vi "AUTON_Index.vi"(0 "Auton Array":dbl[][](array[numeric]), 5 "MeasuredHeading":dbl, 7 "LeftEncoder":dbl, 9 "RightEncoder":dbl, 11 "Harvester DIO":bool) -> (4 "Left Drive":dbl, 6 "Right Drive":dbl, 8 "Indexer":dbl, 10 "Shooter Elevation":dbl, 13 "Flipper":dbl, 14 "Roller":dbl, 15 "Shooter Wheels":dbl)   [LabVIEW 2012]
uses:
  Robot Global Data.vi
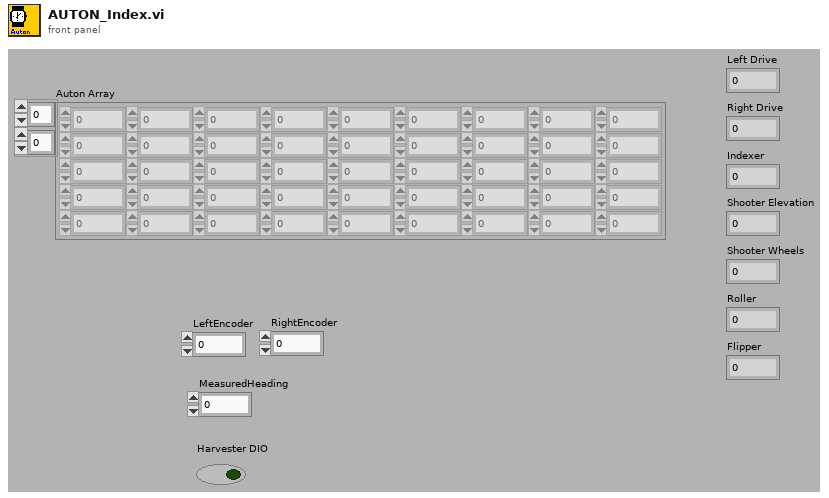
[diagram p1: front panel]
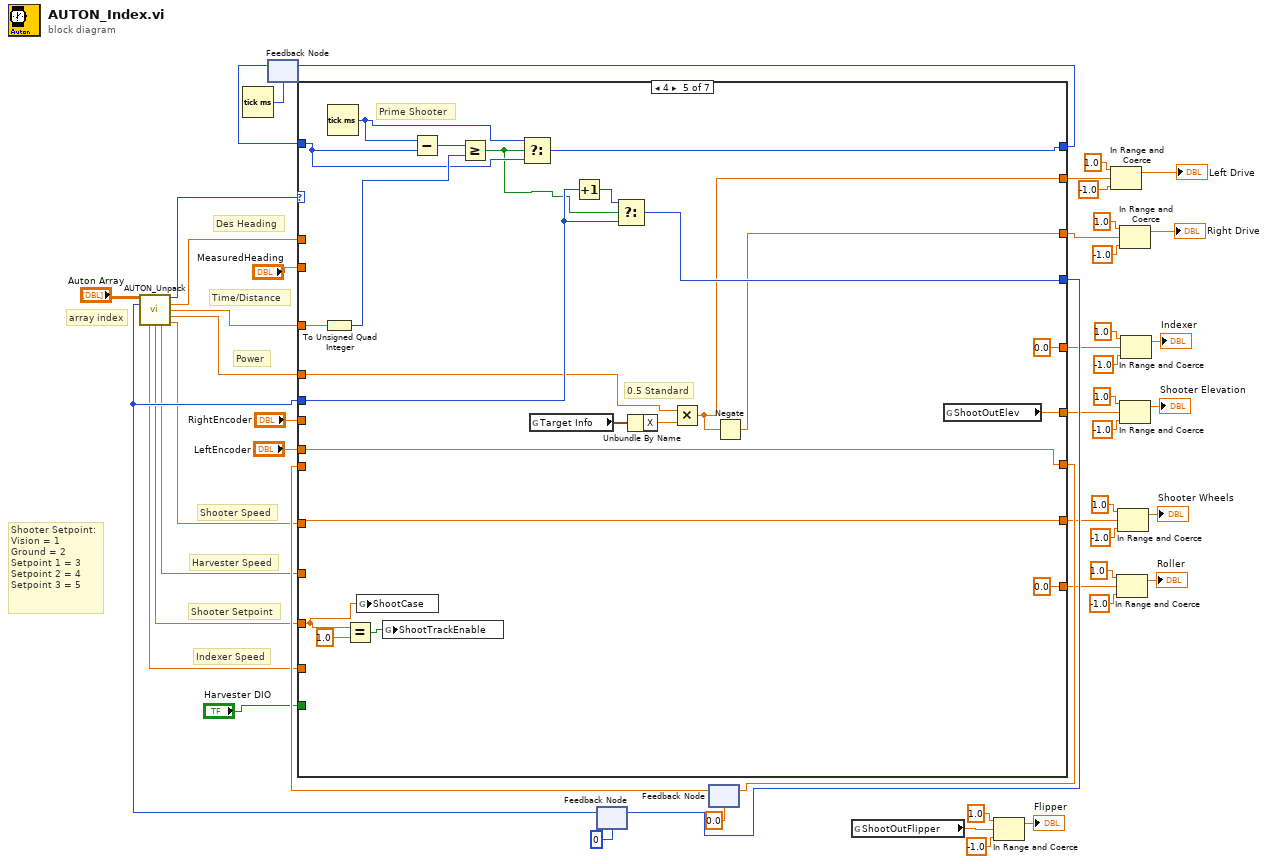
[diagram p0: block diagram]
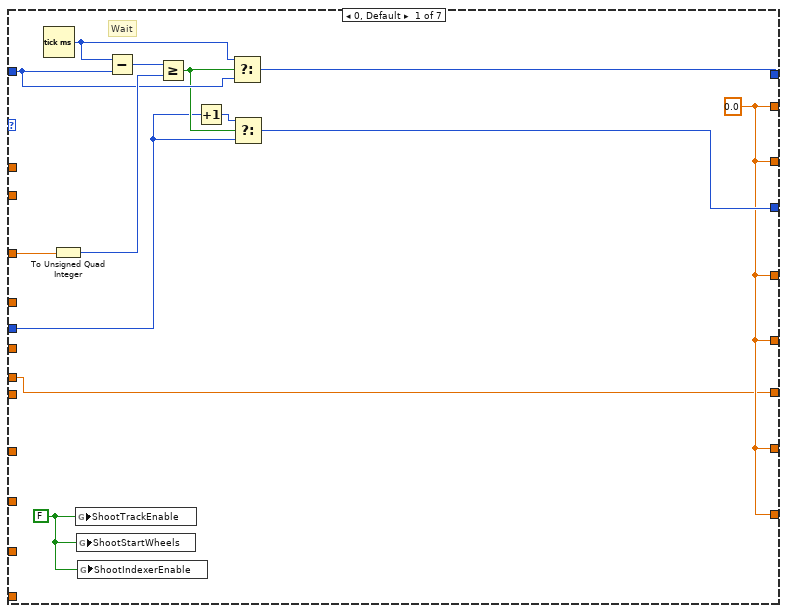
[diagram p2: hidden frame]
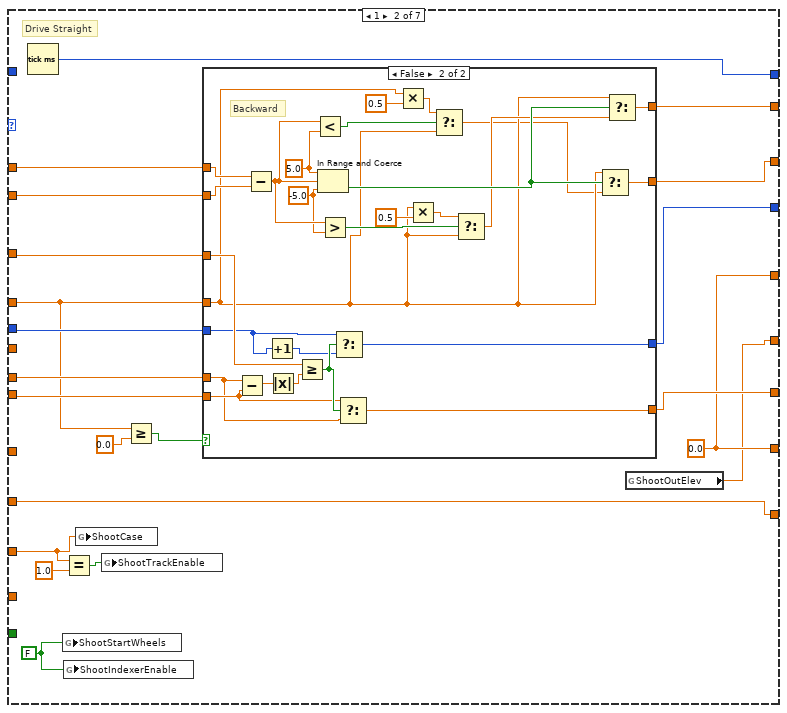
[diagram p3: hidden frame]
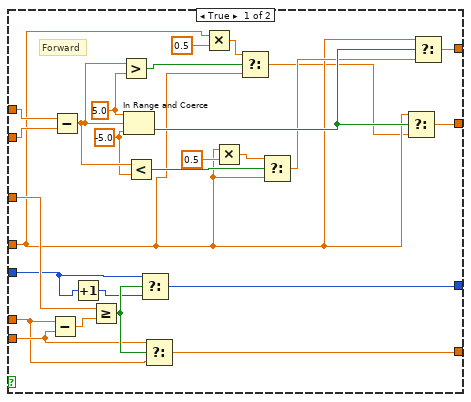
[diagram p4: hidden frame]
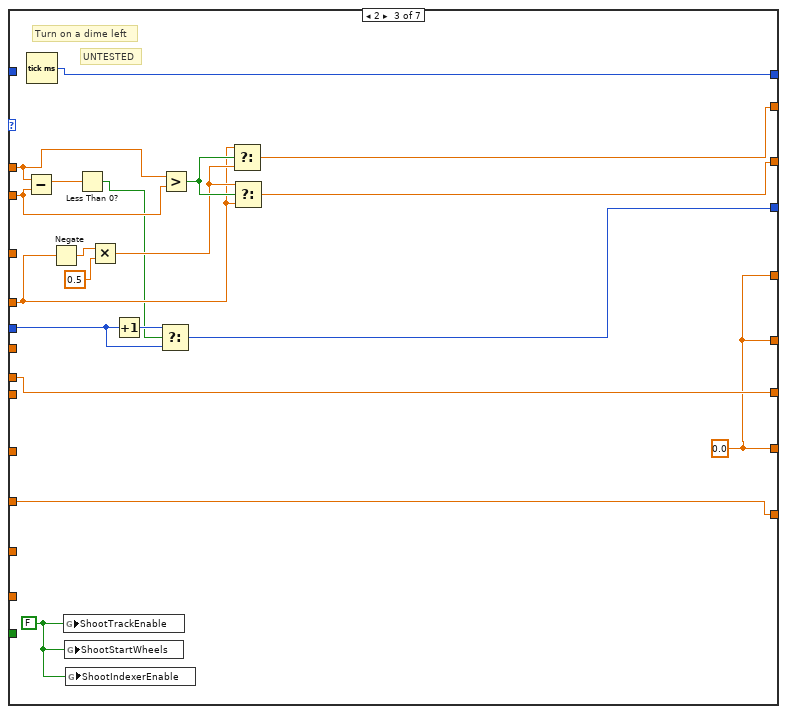
[diagram p5: hidden frame]
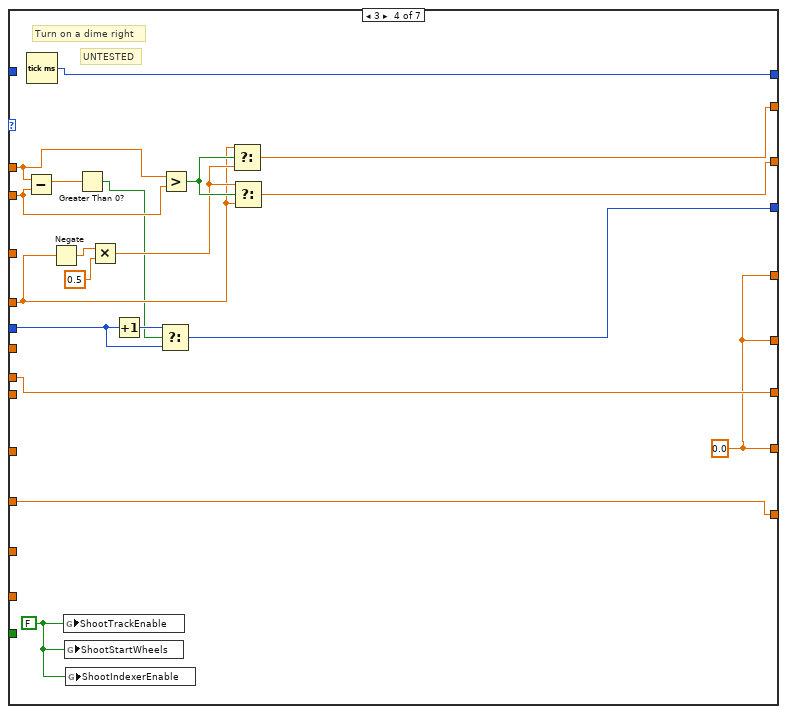
[diagram p6: hidden frame]
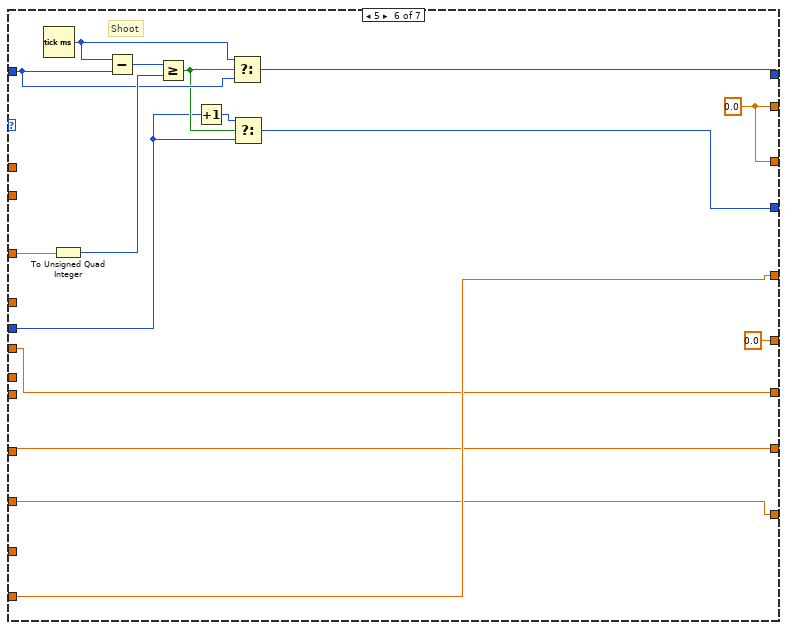
[diagram p7: hidden frame]
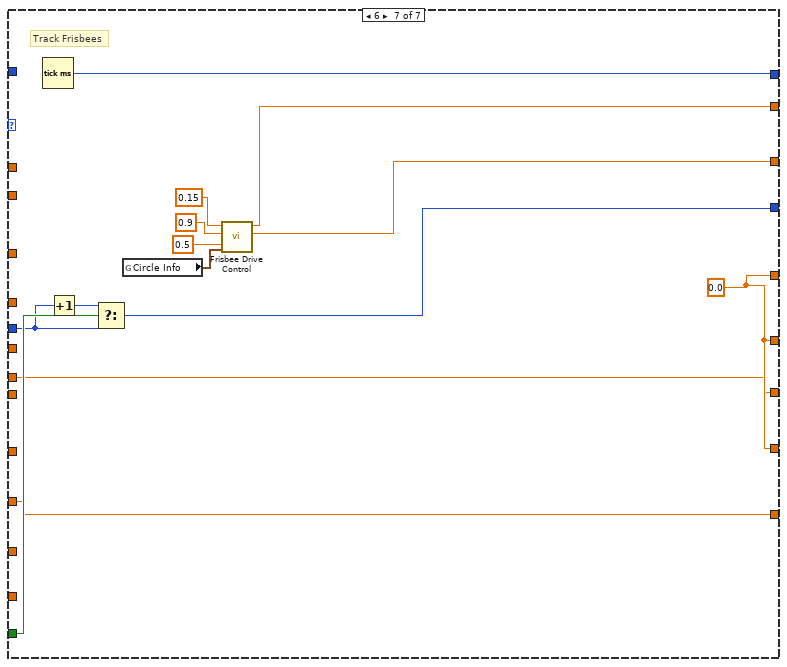
[diagram p8: hidden frame]
diagram:
  # "Shooter Setpoint:\nVision = 1\nGround = 2\nSetpoint 1 = 3\nSetpoint 2 = 4\nSetpoint 3 = 5"
  # "Indexer Speed"
  # "Shooter Speed"
  # "Shooter Setpoint"
  # "Harvester Speed"
  # "Des Heading"
  # "Time/Distance"
  # "Power"
  # "array index"
  n1 = Tick Count (ms)() -> (millisecond timer value=w47:u32)
  n2 = feedback #1(w47) -> (w49:u32)
  n3 = feedback #2(0) -> (w26:i32)
  n4 = call "AUTON_Unpack.vi"("all rows"="Auton Array", "Index"=w26) -> ("Primitive ID"=w30:i16, "Desired Heading"=w28:dbl, "Time/Distance"=w27:dbl, "Power"=w29:dbl, "Indexer Speed"=w22:dbl, "Shooter Setpoint"=w23:dbl, "Harvester Speed"=w24:dbl, "Shooter Speed"=w25:dbl)  [unwired: 6 in]
  n5 = feedback #3(0.0) -> (w32:dbl)
  n6 = case shown="4" w30 {
    tunnel: [w55 w82 w151 w170 w194 w206 w225] -> w35
    tunnel: w26 -> [w56 w77 w154 w173 w185 w207 w227]
    tunnel: [w63 w74 w156 w175 w183 w214 w218] -> w37
    tunnel: w49 -> [w60 _ _ _ w184 w211 _]
    tunnel: w27 -> [w54 w83 _ _ w186 w205 _]
    tunnel: w28 -> [_ w81 w149 w168 _ _ _]
    tunnel: [w53 w79 w152 w171 w177 w204 w220] -> w45
    tunnel: [w53 w78 w153 w172 w176 w204 w219] -> w38
    tunnel: w29 -> [_ w73 w143 w162 w178 _ _]
    tunnel: "LeftEncoder" -> [w51 w75 w150 w169 w198 _ w216]
    tunnel: "MeasuredHeading" -> [_ w80 w148 w167 _ _ _]
    tunnel: "RightEncoder" -> [_ _ _ _ _ w199 _]
    tunnel: w32 -> [_ w76 _ _ _ _ _]
    tunnel: [w51 w84 w150 w169 w198 w199 w216] -> w31
    tunnel: w25 -> [_ _ _ _ w197 w201 _]
    tunnel: w24 -> [_ w68 w140 w159 _ w200 w215]
    tunnel: w23 -> [_ w65 _ _ w190 _ _]
    tunnel: w22 -> [_ _ _ _ _ w203 _]
    tunnel: [w53 w68 w140 w159 0.0 ("Harvester Speed") w200 w215] -> w6
    tunnel: [w53 w70 w141 w160 w197 w201 w217] -> w5
    tunnel: [w53 w64 w141 w160 w182 0.0 ("ShootOutElev") w217] -> w4
    tunnel: [w53 w70 w141 w160 0.0 ("Numeric") w203 w217] -> w3
    tunnel: "Harvester DIO" -> [_ _ _ _ _ _ w228]
    frame 0, Default {
      w52 = FALSE ("ShootTrackEnable")
      w53 = 0.0 ("Numeric")
      # "Wait"
      n7 = Tick Count (ms)() -> (millisecond timer value=w59:u32)
      n8 = To Unsigned Quad Integer(1:w54) -> (0:w61:u64)
      n9 = global write "Robot Global Data.vi" "ShootTrackEnable"(w52) -> ()
      n10 = global write "Robot Global Data.vi" "ShootStartWheels"(w52) -> ()
      n11 = global write "Robot Global Data.vi" "ShootIndexerEnable"(w52) -> ()
      n12 = Subtract(x=w59, y=w60) -> (x-y=w62:u32)
      n13 = Greater Or Equal?(x=w62, y=w61) -> (x >= y?=w58:bool)
      n14 = Increment(x=w56) -> (x+1=w57:i32)
      n15 = Select(t=w59, s=w58, f=w60) -> (s? t:f=w63:u32)
      n16 = Select(t=w57, s=w58, f=w56) -> (s? t:f=w55:i32)
    }
    frame 1 {
      w69 = FALSE ("ShootTrackEnable")
      w70 = 0.0 ("Numeric")
      # "Drive Straight"
      n17 = Tick Count (ms)() -> (millisecond timer value=w74:u32)
      n18 = global write "Robot Global Data.vi" "ShootStartWheels"(w69) -> ()
      n19 = Equal?(x=w65, y=1.0) -> (x = y?=w66:bool)
      n20 = global write "Robot Global Data.vi" "ShootIndexerEnable"(w69) -> ()
      n21 = global write "Robot Global Data.vi" "ShootCase"(w65) -> ()
      n22 = global write "Robot Global Data.vi" "ShootTrackEnable"(w66) -> ()
      n23 = Greater Or Equal?(x=w73, y=0.0) -> (x >= y?=w71:bool)
      n24 = case shown="False" w71 {
        tunnel: [w110 w137] -> w84
        tunnel: w83 -> [w108 w136]
        tunnel: [w106 w134] -> w82
        tunnel: w81 -> [w105 w133]
        tunnel: w80 -> [w104 w132]
        tunnel: [w102 w130] -> w79
        tunnel: [w101 w129] -> w78
        tunnel: w73 -> [w90 w118]
        tunnel: w77 -> [w87 w115]
        tunnel: w76 -> [w86 w114]
        tunnel: w75 -> [w85 w113]
        frame True {
          w98 = -5.0 ("lower limit")
          w100 = 5.0 ("upper limit")
          # "Forward"
          n25 = Subtract(x=w85, y=w86) -> (x-y=w109:dbl)
          n26 = Subtract(x=w105, y=w104) -> (x-y=w99:dbl)
          n27 = Increment(x=w87) -> (x+1=w88:i32)
          n28 = Greater Or Equal?(x=w108, y=w109) -> (x >= y?=w107:bool)
          n29 = Greater?(x=w99, y=w100) -> (0:w93:bool)
          n30 = In Range and Coerce(upper limit=w100, x=w99, lower limit=w98) -> (In Range?=w103:bool)  [unwired: 1 out]
          n31 = Less?(x=w99, y=w98) -> (x < y?=w97:bool)
          n32 = Select(t=w87, s=w107, f=w88) -> (s? t:f=w106:i32)
          n33 = Select(t=w86, s=w107, f=w85) -> (s? t:f=w110:dbl)
          n34 = Multiply(x=w90, y=0.5) -> (x*y=w92:dbl)
          n35 = Multiply(x=w90, y=0.5) -> (x*y=w95:dbl)
          n36 = Select(t=w92, s=w93, f=w90) -> (s? t:f=w89:dbl)
          n37 = Select(t=w95, s=w97, f=w90) -> (s? t:f=w94:dbl)
          n38 = Select(t=w90, s=w103, f=w89) -> (s? t:f=w101:dbl)
          n39 = Select(t=w90, s=w103, f=w94) -> (s? t:f=w102:dbl)
        }
        frame False {
          w126 = -5.0 ("lower limit")
          w128 = 5.0 ("upper limit")
          # "Backward"
          n40 = Subtract(x=w113, y=w114) -> (x-y=w111:dbl)
          n41 = Subtract(x=w133, y=w132) -> (x-y=w127:dbl)
          n42 = Increment(x=w115) -> (x+1=w116:i32)
          n43 = Absolute Value(x=w111) -> (abs(x)=w112:dbl)
          n44 = Greater Or Equal?(x=w136, y=w112) -> (x >= y?=w135:bool)
          n45 = Less?(x=w127, y=w128) -> (x < y?=w121:bool)
          n46 = In Range and Coerce(upper limit=w128, x=w127, lower limit=w126) -> (In Range?=w131:bool)  [unwired: 1 out]
          n47 = Greater?(x=w127, y=w126) -> (0:w125:bool)
          n48 = Select(t=w115, s=w135, f=w116) -> (s? t:f=w134:i32)
          n49 = Select(t=w114, s=w135, f=w113) -> (s? t:f=w137:dbl)
          n50 = Multiply(x=w118, y=0.5) -> (x*y=w120:dbl)
          n51 = Multiply(x=w118, y=0.5) -> (x*y=w123:dbl)
          n52 = Select(t=w120, s=w121, f=w118) -> (s? t:f=w117:dbl)
          n53 = Select(t=w123, s=w125, f=w118) -> (s? t:f=w122:dbl)
          n54 = Select(t=w118, s=w131, f=w117) -> (s? t:f=w129:dbl)
          n55 = Select(t=w118, s=w131, f=w122) -> (s? t:f=w130:dbl)
        }
      }
      n56 = global read "Robot Global Data.vi" "ShootOutElev"() -> (w64:dbl)
    }
    frame 2 {
      w141 = 0.0 ("Numeric")
      w142 = FALSE ("ShootTrackEnable")
      # "UNTESTED"
      # "Turn on a dime left"
      n57 = Subtract(x=w149, y=w148) -> (x-y=w139:dbl)
      n58 = Tick Count (ms)() -> (millisecond timer value=w156:u32)
      n59 = Negate(x=w143) -> (-x=w146:dbl)
      n60 = global write "Robot Global Data.vi" "ShootTrackEnable"(w142) -> ()
      n61 = global write "Robot Global Data.vi" "ShootStartWheels"(w142) -> ()
      n62 = global write "Robot Global Data.vi" "ShootIndexerEnable"(w142) -> ()
      n63 = Less Than 0?(x=w139) -> (x < 0?=w138:bool)
      n64 = Multiply(x=w146, y=0.5) -> (x*y=w144:dbl)
      n65 = Increment(x=w154) -> (x+1=w155:i32)
      n66 = Select(t=w155, s=w138, f=w154) -> (s? t:f=w151:i32)
      n67 = Greater?(x=w149, y=w148) -> (0:w147:bool)
      n68 = Select(t=w143, s=w147, f=w144) -> (s? t:f=w152:dbl)
      n69 = Select(t=w144, s=w147, f=w143) -> (s? t:f=w153:dbl)
    }
    frame 3 {
      w160 = 0.0 ("Numeric")
      w161 = FALSE ("ShootTrackEnable")
      # "UNTESTED"
      # "Turn on a dime right"
      n70 = Subtract(x=w168, y=w167) -> (x-y=w158:dbl)
      n71 = Tick Count (ms)() -> (millisecond timer value=w175:u32)
      n72 = Negate(x=w162) -> (-x=w165:dbl)
      n73 = global write "Robot Global Data.vi" "ShootTrackEnable"(w161) -> ()
      n74 = global write "Robot Global Data.vi" "ShootStartWheels"(w161) -> ()
      n75 = global write "Robot Global Data.vi" "ShootIndexerEnable"(w161) -> ()
      n76 = Greater Than 0?(x=w158) -> (x > 0?=w157:bool)
      n77 = Multiply(x=w165, y=0.5) -> (x*y=w163:dbl)
      n78 = Increment(x=w173) -> (x+1=w174:i32)
      n79 = Select(t=w174, s=w157, f=w173) -> (s? t:f=w170:i32)
      n80 = Greater?(x=w168, y=w167) -> (0:w166:bool)
      n81 = Select(t=w162, s=w166, f=w163) -> (s? t:f=w171:dbl)
      n82 = Select(t=w163, s=w166, f=w162) -> (s? t:f=w172:dbl)
    }
    frame 4 {
      # "0.5 Standard"
      # "Prime Shooter"
      n83 = To Unsigned Quad Integer(1:w186) -> (0:w188:u64)
      n84 = Tick Count (ms)() -> (millisecond timer value=w187:u32)
      n85 = Equal?(x=w190, y=1.0) -> (x = y?=w191:bool)
      n86 = global write "Robot Global Data.vi" "ShootCase"(w190) -> ()
      n87 = global write "Robot Global Data.vi" "ShootTrackEnable"(w191) -> ()
      n88 = Subtract(x=w187, y=w184) -> (x-y=w189:u32)
      n89 = Greater Or Equal?(x=w189, y=w188) -> (x >= y?=w181:bool)
      n90 = Select(t=w187, s=w181, f=w184) -> (s? t:f=w183:u32)
      n91 = global read "Robot Global Data.vi" "Target Info"() -> (w180:cluster{"X":dbl, "Y":dbl, "Distance (ft)":dbl})
      n92 = Increment(x=w185) -> (x+1=w193:i32)
      n93 = Select(t=w193, s=w181, f=w185) -> (s? t:f=w194:i32)
      n94 = Unbundle By Name(w180) -> ("X"=w179:dbl)
      n95 = Multiply(x=w178, y=w179) -> (x*y=w177:dbl)
      n96 = Negate(x=w177) -> (-x=w176:dbl)
      n97 = global read "Robot Global Data.vi" "ShootOutElev"() -> (w182:dbl)
    }
    frame 5 {
      w204 = 0.0 ("Numeric")
      # "Shoot"
      n98 = Tick Count (ms)() -> (millisecond timer value=w210:u32)
      n99 = To Unsigned Quad Integer(1:w205) -> (0:w212:u64)
      n100 = Subtract(x=w210, y=w211) -> (x-y=w213:u32)
      n101 = Greater Or Equal?(x=w213, y=w212) -> (x >= y?=w209:bool)
      n102 = Increment(x=w207) -> (x+1=w208:i32)
      n103 = Select(t=w210, s=w209, f=w211) -> (s? t:f=w214:u32)
      n104 = Select(t=w208, s=w209, f=w207) -> (s? t:f=w206:i32)
    }
    frame 6 {
      w217 = 0.0 ("Indexer Speed")
      # "Track Frisbees"
      n105 = Tick Count (ms)() -> (millisecond timer value=w218:u32)
      n106 = Increment(x=w227) -> (x+1=w226:i32)
      n107 = Select(t=w226, s=w228, f=w227) -> (s? t:f=w225:i32)
      n108 = global read "Robot Global Data.vi" "Circle Info"() -> (w221:cluster{dbl, dbl})
      n109 = call "Frisbee Drive Control.vi"("Circle Info"=w221, "Vertical Constant"=0.5, "Horizontal Constant"=0.9, "Deadband"=0.15) -> ("Right Drive"=w219:dbl, "Left Drive"=w220:dbl)  [unwired: 6 in]
    }
  }
  n110 = feedback-in #1(w37) -> ()
  n111 = feedback-in #2(w35) -> ()
  n112 = feedback-in #3(w31) -> ()
  n113 = global read "Robot Global Data.vi" "ShootOutFlipper"() -> (w2:dbl)
  n114 = In Range and Coerce(upper limit=1.0, x=w2, lower limit=-1.0) -> (coerced(x)=→"Flipper":dbl)  [unwired: 1 out]
  n115 = In Range and Coerce(upper limit=1.0, x=w45, lower limit=-1.0) -> (coerced(x)=→"Left Drive":dbl)  [unwired: 1 out]
  n116 = In Range and Coerce(upper limit=1.0, x=w6, lower limit=-1.0) -> (coerced(x)=→"Roller":dbl)  [unwired: 1 out]
  n117 = In Range and Coerce(upper limit=1.0, x=w5, lower limit=-1.0) -> (coerced(x)=→"Shooter Wheels":dbl)  [unwired: 1 out]
  n118 = In Range and Coerce(upper limit=1.0, x=w38, lower limit=-1.0) -> (coerced(x)=→"Right Drive":dbl)  [unwired: 1 out]
  n119 = In Range and Coerce(upper limit=1.0, x=w4, lower limit=-1.0) -> (coerced(x)=→"Shooter Elevation":dbl)  [unwired: 1 out]
  n120 = In Range and Coerce(upper limit=1.0, x=w3, lower limit=-1.0) -> (coerced(x)=→"Indexer":dbl)  [unwired: 1 out]
